vi "VCI_CAN_OBJ_CONVERT.vi"(1 "VCI_CAN_OBJ":T2) -> (0 "VCI_CAN_OBJ_1":T1)   [LabVIEW 2018, in "ControlCan.lvlib"]
uses:
  ControlCan.lvlib
  VCI_CAN_OBJ.ctl
  VCI_CAN_OBJ_1.ctl
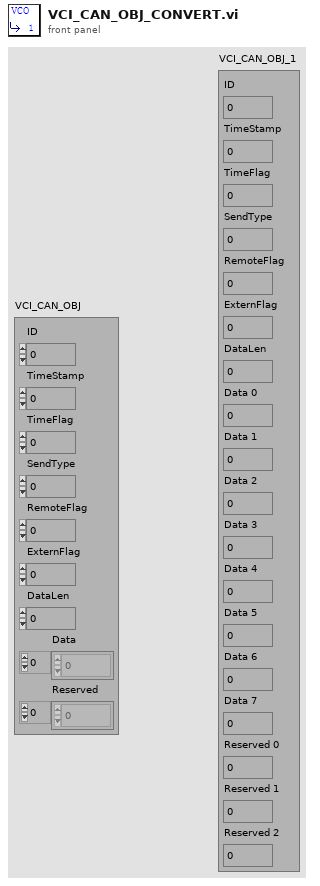
[diagram p1: front panel]
types:
  T1 = typedef "ControlCAN.lvlib/VCI_CAN_OBJ_1.ctl" = cluster{"ID":u32, "TimeStamp":u32, "TimeFlag":u8, "SendType":u8, "RemoteFlag":u8, "ExternFlag":u8, "DataLen":u8, "Data 0":u8, "Data 1":u8, "Data 2":u8, "Data 3":u8, "Data 4":u8, "Data 5":u8, "Data 6":u8, "Data 7":u8, "Reserved 0":u8, "Reserved 1":u8, "Reserved 2":u8}
  T2 = typedef "ControlCAN.lvlib/VCI_CAN_OBJ.ctl" = cluster{"ID":u32, "TimeStamp":u32, "TimeFlag":u8, "SendType":u8, "RemoteFlag":u8, "ExternFlag":u8, "DataLen":u8, "Data":u8[], "Reserved":u8[]}
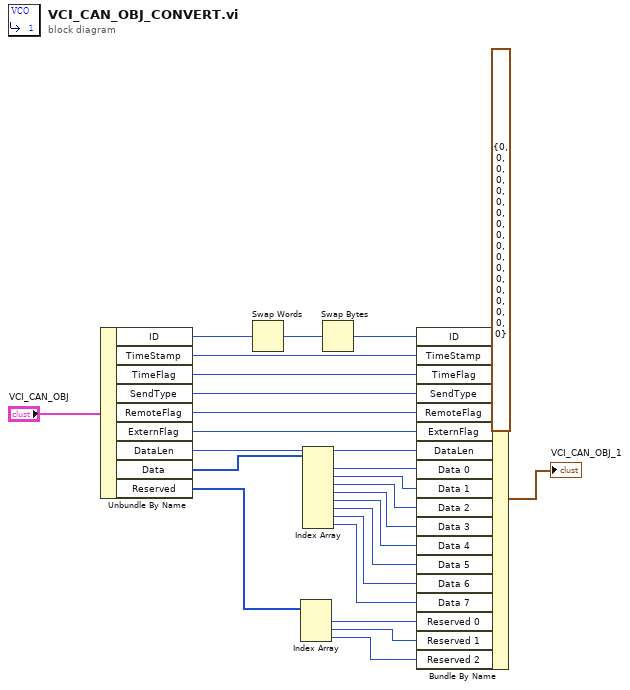
[diagram p0: block diagram]
diagram:
  n1 = Unbundle By Name("VCI_CAN_OBJ") -> ("ID"=w2:u32, "TimeStamp"=w23:u32, "TimeFlag"=w22:u8, "SendType"=w21:u8, "RemoteFlag"=w20:u8, "ExternFlag"=w4:u8, "DataLen"=w19:u8, "Data"=w18:u8[], "Reserved"=w9:u8[])
  n2 = Swap Words(1:w2) -> (0:w3:u32)
  n3 = Index Array(array=w9) -> (element #1=w8:u8, element #2=w7:u8, element #3=w6:u8)  [unwired: 3 in]
  n4 = Index Array(array=w18) -> (element #1=w17:u8, element #2=w16:u8, element #3=w15:u8, element #4=w14:u8, element #5=w13:u8, element #6=w12:u8, element #7=w11:u8, element #8=w10:u8)  [unwired: 8 in]
  n5 = Swap Bytes(anything=w3) -> (byte swapped=w1:u32)
  n6 = Bundle By Name(cluster=T1 {"ID"=0, "TimeStamp"=0, "TimeFlag"=0, "SendType"=0, "RemoteFlag"=0, "ExternFlag"=0, "DataLen"=0, "Data 0"=0, "Data 1"=0, "Data 2"=0, "Data 3"=0, "Data 4"=0, "Data 5"=0, "Data 6"=0, "Data 7"=0, "Reserved 0"=0, "Reserved 1"=0, "Reserved 2"=0} ("VCI_CAN_OBJ_1"), "ID"=w1, "TimeStamp"=w23, "TimeFlag"=w22, "SendType"=w21, "RemoteFlag"=w20, "ExternFlag"=w4, "DataLen"=w19, "Data 0"=w17, "Data 1"=w16, "Data 2"=w15, "Data 3"=w14, "Data 4"=w13, "Data 5"=w12, "Data 6"=w11, "Data 7"=w10, "Reserved 0"=w8, "Reserved 1"=w7, "Reserved 2"=w6) -> (→"VCI_CAN_OBJ_1":T1)
